vi "offset.vi"(1 "coordinates (in)":T1 {"element" format="%.2f"; "element" format="%.2f"; "element" format="%.2f"}, 2 "set?":bool, 3 "offset":cluster{dbl, dbl, dbl} {"?" format="%.2f"; "?" format="%.2f"; "?" format="%.2f"}) -> (0 "coordinates (out)":cluster{dbl, dbl, dbl} {"?" format="%.2f"; "?" format="%.2f"; "?" format="%.2f"})   [LabVIEW 2009]
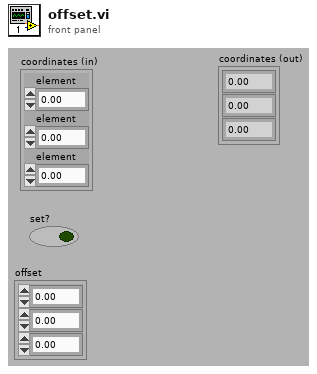
[diagram p1: front panel]
types:
  T1 = cluster{"element":dbl, "element":dbl, "element":dbl}
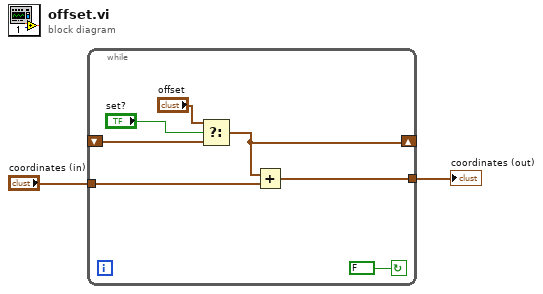
[diagram p0: block diagram]
diagram:
  n1 = while {
    tunnel: "coordinates (in)" -> [w9]
    tunnel: [w8] -> w1
    shift-right: [w4] -> _
    shift-left: _ -> [w5]
    stop <- FALSE continue-if-true
    n2 = Select(t="offset", s="set?", f=w5) -> (s? t:f=w4:cluster{dbl, dbl, dbl})
    n3 = Add(x=w4, y=w9) -> (x+y=w8:cluster{dbl, dbl, dbl})
  }
  "coordinates (out)" <- w1
